vi "Initialize.vi"(8 "error in (no error)":errorcluster, 11 "OD600 in":refnum<class "OD600.lvclass">) -> (0 "error out":errorcluster, 3 "OD600 out":refnum<class "OD600.lvclass">)   [LabVIEW 2013, in "OD600.lvlib" / "OD600.lvclass"]
uses:
  OD600.lvclass
  <vilib>/Instr/_visa.llb/VISA Flush IO Buffer Mask.ctl
  OD600.lvclass/OD600.ctl
  Read OD600.vi
  Read Sampling Interval.vi
  Write VISA 1.vi
  <vilib>/Instr/_visa.llb/VISA Configure Serial Port (Instr).vi
  PluginInterface/PluginInterface.lvlibp/PluginInterfaceClass/Read Name.vi
  PluginInterface/PluginInterface.lvlibp/PluginInterfaceClass/Read TDMS File Path.vi
  PluginInterface/PluginInterface.lvlibp/PluginInterfaceClass/Read DVR.vi
  PluginInterface/PluginInterface.lvlibp/PluginInterfaceClass/Write TDMS.vi
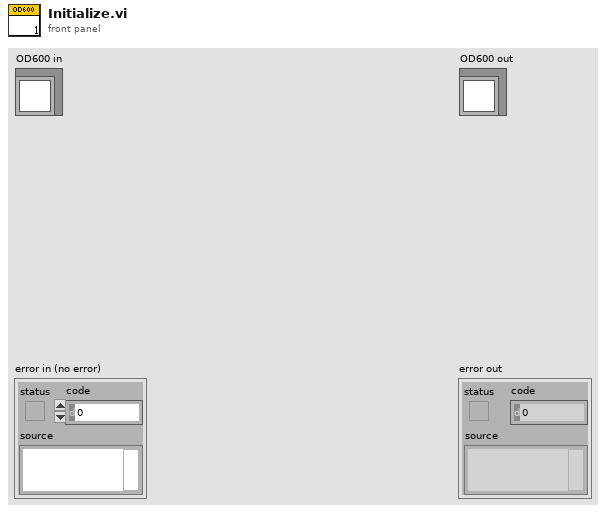
[diagram p1: front panel]
types:
  T1 = enum16{"open", "open or create", "create or replace", "create", "open (read-only)"}
  T2 = typedef "VISA Flush IO Buffer Mask.ctl" = u16
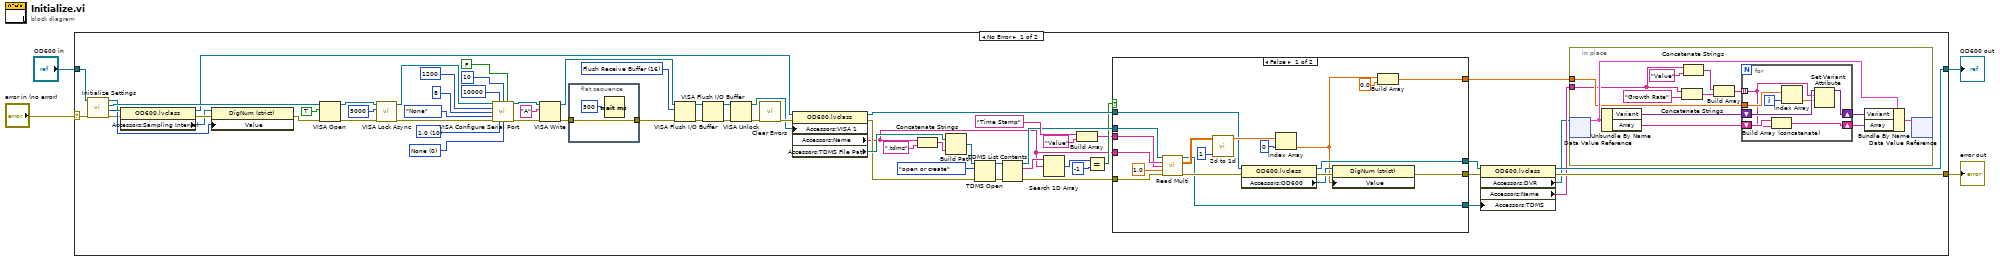
[diagram p0: block diagram]
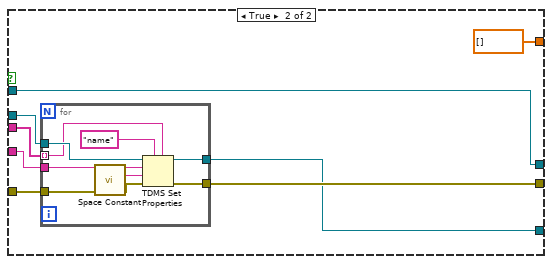
[diagram p2: hidden frame]
diagram:
  n1 = case shown="No Error" "error in (no error)" {
    selector: "error in (no error)" -> [w51 w129]
    tunnel: [w37 w129] -> w2
    tunnel: [w39 w128] -> w1
    tunnel: "OD600 in" -> [w35 w128]
    frame No Error {
      w56 = T2 16 items=["Flush Receive Buffer"=16, "Write Transmit Buffer to Device"=32, "Flush Receive Buffer (No I/O)"=64, "Flush Transmit Buffer"=128] ("Mask")
      w59 = u16 0 items=["None", "XON/XOFF", "RTS/CTS", "XON/XOFF & RTS/CTS", "DTR/DSR", "XON/XOFF & DTR/DSR"] ("flow control (0:none)")
      w60 = u16 10 items=["1.0"=10, "1.5"=15, "2.0"=20] ("stop bits (10: 1 bit)")
      n2 = call "Initialize Settings.vi"("error in (no error)"=w51, "OD600 in"=w35) -> ("error out"=w27:errorcluster, "Sampling Interval 2"=w29:i32, "VISA out"=w34:refnum<visa-resource-name>, "OD600 out"=w32:refnum<class "OD600.lvclass">)  [unwired: 5 in]
      n3 = property class="OD600.lvclass"(reference=w32, error in=w27) -> (reference out=w31:refnum<class "OD600.lvclass">, error out=w33:errorcluster, "Accessors:Sampling Interval"=w30:refnum<vi>)
      n4 = property class="DigNum (strict)"(reference=w30, error in=w33, "Value"=w29) -> (error out=w28:errorcluster)  [unwired: 1 out]
      n5 = VISA Open(duplicate session (F)=TRUE, error in (no error)=w28, VISA resource name=w34) -> (VISA resource name=w49:refnum<visa-resource-name>, error out=w48:errorcluster)  [unwired: 2 in]
      n6 = call <vilib>:"VISA Lock Async.vi"("error in (no error)"=w48, "timeout (0)"=u32 5000, "VISA resource name"=w49) -> ("error out"=w45:errorcluster, "VISA resource name out"=w46:refnum<visa-resource-name>)  [unwired: 6 in, 1 out]
      n7 = call-poly "VISA Configure Serial Port"("VISA resource name"=w46, "timeout (10sec)"=u32 10000, "termination char\n(0xA = '\\n' = LF)"=u8 10 ("termination char\n(0xA = '\\n' = LF)"), "Enable Termination\nChar (T)"=FALSE ("Enable Termination\nChar (T)"), "baud rate (9600)"=u32 1200, "data bits (8)"=u16 8, "parity (0:none)"=enum16{"None", "Odd", "Even", "Mark", "Space"}."None", "error in (no error)"=w45, "stop bits (10: 1 bit)"=w60, "flow control (0:none)"=w59) -> ("VISA resource name out"=w55:refnum<visa-resource-name>, "error out"=w54:errorcluster)  [unwired: 4 in]
      n8 = VISA Write(VISA resource name=w55, write buffer="A", error in (no error)=w54) -> (VISA resource name out=w57:refnum<visa-resource-name>, error out=w65:errorcluster)  [unwired: 1 out]
      n9 = flat-sequence {
        tunnel: [w91] -> w58
        tunnel: w65 -> [w91]
        frame #0 {
          n10 = Wait (ms)(milliseconds to wait=u32 500) -> ()  [unwired: 1 out]
        }
      }
      n11 = VISA Flush I/O Buffer(VISA resource name=w57, mask (16)=w56, error in (no error)=w58) -> (VISA resource name out=w52:refnum<visa-resource-name>, error out=w53:errorcluster)
      n12 = VISA Flush I/O Buffer(VISA resource name=w52, error in (no error)=w53) -> (VISA resource name out=w44:refnum<visa-resource-name>, error out=w42:errorcluster)  [unwired: 1 in]
      n13 = VISA Unlock(8:w42, 11:w44) -> (0:w41:errorcluster, 3:w43:refnum<visa-resource-name>)
      n14 = call <vilib>:"Clear Errors.vi"("error in (no error)"=w41) -> ("error out"=w69:errorcluster)  [unwired: 6 in]
      n15 = property class="OD600.lvclass"(reference=w31, error in=w69, "Accessors:VISA 1"=w43) -> (reference out=w13:refnum<class "OD600.lvclass">, error out=w14:errorcluster, "Accessors:Name"=w8:string, "Accessors:TDMS File Path"=w15:path)
      n16 = Concatenate Strings(w8, ".tdms" ("name or relative path")) -> (w16:string)
      n17 = Build Path(base path=w15, name or relative path=w16) -> (appended path=w21:path)
      n18 = TDMS Open(8:w14, 10:T1."open or create" ("operation (0:open)"), 11:w21) -> (0:w20:errorcluster, 3:w18:refnum<k34>)  [unwired: 4 in]
      n19 = TDMS List Contents(4:w20, 7:w18) -> (0:w11:errorcluster, 2:w24:string[], 3:w12:refnum<k34>)  [unwired: 1 in, 1 out]
      n20 = Search 1D Array(1D array=w24, element=w8) -> (index of element=w25:i32)  [unwired: 1 in]
      n21 = Build Array("Time Stamp" ("Channel"), "Value" ("string")) -> (w9:string[])
      n22 = Equal?(x=w25, y=-1) -> (x = y?=w10:bool)
      n23 = case shown="False" w10 {
        tunnel: w12 -> [w101 w119]
        tunnel: [w102 w115] -> w38
        tunnel: w11 -> [w103 w117]
        tunnel: w8 -> [w100 w118]
        tunnel: w13 -> [w99 w114]
        tunnel: w9 -> [w97 w116]
        tunnel: [w98 w114] -> w40
        tunnel: [w94 dbl[] []] -> w6
        tunnel: [w96 w113] -> w36
        frame False {
          n24 = call "Read Multi.vi"("tdms file in"=w101, "group"=w100, "Channel"=w97, "Numeric"=1.0, "error in (no error)"=w103) -> ("tdms file out"=w96:refnum<k34>, "Array"=w108:dbl[][], "error out"=w111:errorcluster)  [unwired: 7 in, 1 out]
          n25 = call "2d to 1d.vi"("index"=1, "array"=w108) -> ("output array"=w107:dbl[])  [unwired: 9 in]
          n26 = property class="OD600.lvclass"(reference=w99, error in=w111) -> (reference out=w98:refnum<class "OD600.lvclass">, error out=w106:errorcluster, "Accessors:OD600"=w105:refnum<vi>)
          n27 = Index Array(array=w107, index=0) -> (element=w95:dbl)
          n28 = property class="DigNum (strict)"(reference=w105, error in=w106, "Value"=w95) -> (error out=w102:errorcluster)  [unwired: 1 out]
          n29 = Build Array(w95, 0.0 ("element")) -> (w94:dbl[])
        }
        frame True {
          n30 = for {
            tunnel: w117 -> [w127]
            tunnel: [w126] -> w115
            tunnel: w119 -> [w125]
            tunnel: w118 -> [w124]
            tunnel: w116 -> [w123] mode=indexing
            tunnel: [w120] -> w113
            n31 = call <vilib>:"Space Constant.vi"() -> ("String"=w121:string)
            n32 = TDMS Set Properties(5:w123, 7:"name" ("property names"), 8:w127, 9:w121, 10:w124, 11:w125) -> (0:w126:errorcluster, 3:w120:refnum<k34>)  [unwired: 2 out]
          }
        }
      }
      n33 = property class="OD600.lvclass"(reference=w40, error in=w38, "Accessors:TDMS"=w36) -> (reference out=w39:refnum<class "OD600.lvclass">, error out=w37:errorcluster, "Accessors:DVR"=w5:refnum<data-value>, "Accessors:Name"=w7:string)
      n34 = in-place {
        in-place-border: w6 -> [w77]
        in-place-border: w7 -> [w74]
        n35 = in-place-dvr #1(w5) -> (w79:cluster{"Array":string[], "Variant":variant})  [unwired: 1 out]
        n36 = Unbundle By Name(w79) -> ("Variant"=w81:variant, "Array"=w71:string[])
        n37 = Concatenate Strings(w74, "Growth Rate" ("string")) -> (w72:string)
        n38 = Concatenate Strings(w74, "Value" ("string")) -> (w73:string)
        n39 = Build Array(w73, w72) -> (w78:string[])
        n40 = for {
          tunnel: w78 -> [w84] mode=indexing
          tunnel: w77 -> [w87]
          shift-right: [w89] -> w80
          shift-left: w81 -> [w90]
          shift-right: [w83] -> w70
          shift-left: w71 -> [w85]
          i -> [w88]
          n41 = Build Array (concatenate)(w85, w84) -> (w83:string[])
          n42 = Index Array(array=w87, index=w88) -> (element=w86:dbl)
          n43 = Set Variant Attribute(Variant=w90, name=w84, value=w86) -> (Variant out=w89:variant)  [unwired: 1 in, 2 out]
        }
        n44 = Bundle By Name(cluster=w79, "Variant"=w80, "Array"=w70) -> (w82:cluster{"Array":string[], "Variant":variant})
        n45 = in-place-dvr #1(w82) -> ()  [unwired: 2 out]
      }
    }
    frame Error {
    }
  }
  "error out" <- w2
  "OD600 out" <- w1
